vi "Initialize.vi"(6 "error in":errorcluster) -> (0 "error out":errorcluster, 3 "VISA resource name out":refnum<visa-resource-name>)   [LabVIEW 2023, in "Aim TTi 1908P DMM.lvlib"]
uses:
  Aim TTi 1908P DMM.lvlib
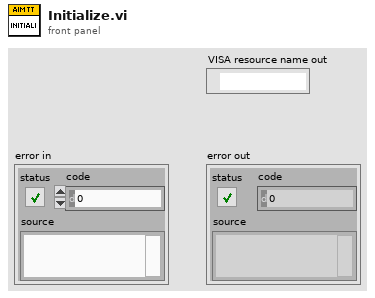
[diagram p1: front panel]
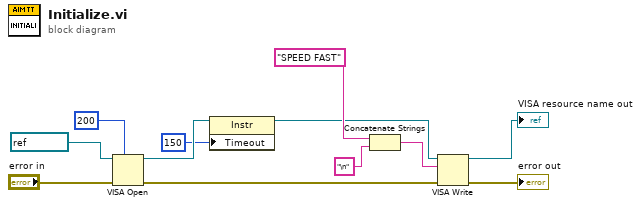
[diagram p0: block diagram]
diagram:
  n1 = VISA Open(timeout (0)=u32 200 ("VISA Open timeout (0)"), error in (no error)="error in", VISA resource name=refnum<visa-resource-name> "DMM") -> (VISA resource name=w9:refnum<visa-resource-name>, error out=w4:errorcluster)  [unwired: 2 in]
  n2 = property class="Instr"(reference=w9, "Timeout"=u32 150 ("General Settings:Timeout Value")) -> (reference out=w2:refnum<visa-resource-name>)  [unwired: 1 in, 1 out]
  n3 = Concatenate Strings("SPEED FAST" ("Read command"), "\n" ("string")) -> (w6:string)
  n4 = VISA Write(VISA resource name=w2, write buffer=w6, error in (no error)=w4) -> (VISA resource name out=→"VISA resource name out":refnum<visa-resource-name>, error out=→"error out":errorcluster)  [unwired: 1 out]
